vi "GUI Monitoring Graph Window.vi"(4 "Graph Unit":string, 6 "Window Title":string, 8 "BPM?":bool, 9 "Monitoring Queue Name":string, 10 "Selected Readings":u32[](array[numeric])=[0, 1, 2, 3, 4, 5, 6, 7, 8, 9, 10, 11, 12, 13, 14, 15, 16, 17, 18, 19, 20, 21, 22, 23, 24, 25, 26, 27, 28, 29, 30, 31, 32, 33, 34, 35], 11 "Variable Names":string[](array[string])=["ACH01B", "ACH02", "ACH03A", "ACH03B", "ACH04", "ACH05A", "ACH05B", "ACH06", "ACH07A", "ACH07B", "ACH08", "ACH09A", "ACH09B", "ACH10", "ACH11A", "ACH11B", "ACH12", "ACH01A"]) -> ()   [LabVIEW 2011, in "User Interface Window VIs.lvlib"]
uses:
  User Interface Window VIs.lvlib
  Types Definitions/Type Monitoring Sample.ctl
  <vilib>/Platform/TimedLoop/XDataNode/timing_clust.ctl
  <vilib>/Platform/TimedLoop/XDataNode/nitl_modes.ctl
  <vilib>/Platform/TimedLoop/XDataNode/wakeup.ctl
  <vilib>/express/express shared/transition.llb/Dynamic To Waveform Array.vi
  <vilib>/express/express signal manip/GetorSetDDTAttributes/Set DDT Attributes/SetT0.vi
  <vilib>/express/express shared/transition.llb/Waveform Array To Dynamic.vi
  <vilib>/Platform/TimedLoop/XDataNode/XDataNode.xnode
  <vilib>/express/express signal manip/GetorSetDDTAttributes/Set DDT Attributes/Set DDT Properties.xnode
  Common VIs.lvlib
  <vilib>/Platform/TimedLoop/XDataNode/XDNodeRunTimeDep.lvlib
  User Interface VIs.lvlib
  Type Definitions.lvlib
panel:
  out "Time Stamp on FOFB Controller":timestamp caption="Data/Hora Atual no\nControlador do FOFB"
  out "error out":errorcluster
  in  "All/None":bool=TRUE caption="Todos/Nenhum"
  out "Graph":dynamicdata(graph)=[{"t0"=timestamp(3440556827.6210413 s since 1904-01-01), "dt"=1.0, "Y"=[0.004733479817708333], "attributes"=variant("NI_ExpTimeStamp"=variant(timestamp timestamp(3440556827.6210413 s since 1904-01-01)))}, {"t0"=timestamp(3440556827.6210413 s since 1904-01-01), "dt"=1.0, "Y"=[0.004206909179687498], "attributes"=variant("NI_ExpTimeStamp"=variant(timestamp timestamp(3440556827.6210413 s since 1904-01-01)))}, {"t0"=timestamp(3440556827.6210413 s since 1904-01-01), "dt"=1.0, "Y"=[-10.43072509765625], "attributes"=variant("NI_ExpTimeStamp"=variant(timestamp timestamp(3440556827.6210413 s since 1904-01-01)))}, {"t0"=timestamp(3440556827.6210413 s since 1904-01-01), "dt"=1.0, "Y"=[-10.430725128173831], "attributes"=variant("NI_ExpTimeStamp"=variant(timestamp timestamp(3440556827.6210413 s since 1904-01-01)))}, {"t0"=timestamp(3440556827.6210413 s since 1904-01-01), "dt"=1.0, "Y"=[0.010971476236979166], "attributes"=variant("NI_ExpTimeStamp"=variant(timestamp timestamp(3440556827.6210413 s since 1904-01-01)))}, {"t0"=timestamp(3440556827.6210413 s since 1904-01-01), "dt"=1.0, "Y"=[0.01062655639648437], "attributes"=variant("NI_ExpTimeStamp"=variant(timestamp timestamp(3440556827.6210413 s since 1904-01-01)))}, {"t0"=timestamp(3440556827.6210413 s since 1904-01-01), "dt"=1.0, "Y"=[0.006206461588541667], "attributes"=variant("NI_ExpTimeStamp"=variant(timestamp timestamp(3440556827.6210413 s since 1904-01-01)))}, {"t0"=timestamp(3440556827.6210413 s since 1904-01-01), "dt"=1.0, "Y"=[0.0061141052246093735], "attributes"=variant("NI_ExpTimeStamp"=variant(timestamp timestamp(3440556827.6210413 s since 1904-01-01)))}, {"t0"=timestamp(3440556827.6210413 s since 1904-01-01), "dt"=1.0, "Y"=[-10.42022705078125], "attributes"=variant("NI_ExpTimeStamp"=variant(timestamp timestamp(3440556827.6210413 s since 1904-01-01)))}, {"t0"=timestamp(3440556827.6210413 s since 1904-01-01), "dt"=1.0, "Y"=[-10.42022705078125], "attributes"=variant("NI_ExpTimeStamp"=variant(timestamp timestamp(3440556827.6210413 s since 1904-01-01)))}, {"t0"=timestamp(3440556827.6210413 s since 1904-01-01), "dt"=1.0, "Y"=[-10.37188720703125], "attributes"=variant("NI_ExpTimeStamp"=variant(timestamp timestamp(3440556827.6210413 s since 1904-01-01)))}, {"t0"=timestamp(3440556827.6210413 s since 1904-01-01), "dt"=1.0, "Y"=[-10.37188720703125], "attributes"=variant("NI_ExpTimeStamp"=variant(timestamp timestamp(3440556827.6210413 s since 1904-01-01)))}, {"t0"=timestamp(3440556827.6210413 s since 1904-01-01), "dt"=1.0, "Y"=[0.0069844563802083336], "attributes"=variant("NI_ExpTimeStamp"=variant(timestamp timestamp(3440556827.6210413 s since 1904-01-01)))}, {"t0"=timestamp(3440556827.6210413 s since 1904-01-01), "dt"=1.0, "Y"=[0.007014038085937505], "attributes"=variant("NI_ExpTimeStamp"=variant(timestamp timestamp(3440556827.6210413 s since 1904-01-01)))}, {"t0"=timestamp(3440556827.6210413 s since 1904-01-01), "dt"=1.0, "Y"=[0.0], "attributes"=variant("NI_ExpTimeStamp"=variant(timestamp timestamp(3440556827.6210413 s since 1904-01-01)))}, {"t0"=timestamp(3440556827.6210413 s since 1904-01-01), "dt"=1.0, "Y"=[0.0], "attributes"=variant("NI_ExpTimeStamp"=variant(timestamp timestamp(3440556827.6210413 s since 1904-01-01)))}, {"t0"=timestamp(3440556827.6210413 s since 1904-01-01), "dt"=1.0, "Y"=[0.0], "attributes"=variant("NI_ExpTimeStamp"=variant(timestamp timestamp(3440556827.6210413 s since 1904-01-01)))}, {"t0"=timestamp(3440556827.6210413 s since 1904-01-01), "dt"=1.0, "Y"=[0.0], "attributes"=variant("NI_ExpTimeStamp"=variant(timestamp timestamp(3440556827.6210413 s since 1904-01-01)))}, {"t0"=timestamp(3440556827.6210413 s since 1904-01-01), "dt"=1.0, "Y"=[0.0], "attributes"=variant("NI_ExpTimeStamp"=variant(timestamp timestamp(3440556827.6210413 s since 1904-01-01)))}, {"t0"=timestamp(3440556827.6210413 s since 1904-01-01), "dt"=1.0, "Y"=[0.0], "attributes"=variant("NI_ExpTimeStamp"=variant(timestamp timestamp(3440556827.6210413 s since 1904-01-01)))}, {"t0"=timestamp(3440556827.6210413 s since 1904-01-01), "dt"=1.0, "Y"=[0.0], "attributes"=variant("NI_ExpTimeStamp"=variant(timestamp timestamp(3440556827.6210413 s since 1904-01-01)))}, {"t0"=timestamp(3440556827.6210413 s since 1904-01-01), "dt"=1.0, "Y"=[0.0], "attributes"=variant("NI_ExpTimeStamp"=variant(timestamp timestamp(3440556827.6210413 s since 1904-01-01)))}, {"t0"=timestamp(3440556827.6210413 s since 1904-01-01), "dt"=1.0, "Y"=[0.0], "attributes"=variant("NI_ExpTimeStamp"=variant(timestamp timestamp(3440556827.6210413 s since 1904-01-01)))}, {"t0"=timestamp(3440556827.6210413 s since 1904-01-01), "dt"=1.0, "Y"=[0.0], "attributes"=variant("NI_ExpTimeStamp"=variant(timestamp timestamp(3440556827.6210413 s since 1904-01-01)))}, {"t0"=timestamp(3440556827.6210413 s since 1904-01-01), "dt"=1.0, "Y"=[0.0], "attributes"=variant("NI_ExpTimeStamp"=variant(timestamp timestamp(3440556827.6210413 s since 1904-01-01)))}, {"t0"=timestamp(3440556827.6210413 s since 1904-01-01), "dt"=1.0, "Y"=[0.0], "attributes"=variant("NI_ExpTimeStamp"=variant(timestamp timestamp(3440556827.6210413 s since 1904-01-01)))}, {"t0"=timestamp(3440556827.6210413 s since 1904-01-01), "dt"=1.0, "Y"=[0.0], "attributes"=variant("NI_ExpTimeStamp"=variant(timestamp timestamp(3440556827.6210413 s since 1904-01-01)))}, {"t0"=timestamp(3440556827.6210413 s since 1904-01-01), "dt"=1.0, "Y"=[0.0], "attributes"=variant("NI_ExpTimeStamp"=variant(timestamp timestamp(3440556827.6210413 s since 1904-01-01)))}, {"t0"=timestamp(3440556827.6210413 s since 1904-01-01), "dt"=1.0, "Y"=[0.0], "attributes"=variant("NI_ExpTimeStamp"=variant(timestamp timestamp(3440556827.6210413 s since 1904-01-01)))}, {"t0"=timestamp(3440556827.6210413 s since 1904-01-01), "dt"=1.0, "Y"=[0.0], "attributes"=variant("NI_ExpTimeStamp"=variant(timestamp timestamp(3440556827.6210413 s since 1904-01-01)))}, {"t0"=timestamp(3440556827.6210413 s since 1904-01-01), "dt"=1.0, "Y"=[0.0], "attributes"=variant("NI_ExpTimeStamp"=variant(timestamp timestamp(3440556827.6210413 s since 1904-01-01)))}, {"t0"=timestamp(3440556827.6210413 s since 1904-01-01), "dt"=1.0, "Y"=[0.0], "attributes"=variant("NI_ExpTimeStamp"=variant(timestamp timestamp(3440556827.6210413 s since 1904-01-01)))}, {"t0"=timestamp(3440556827.6210413 s since 1904-01-01), "dt"=1.0, "Y"=[0.0], "attributes"=variant("NI_ExpTimeStamp"=variant(timestamp timestamp(3440556827.6210413 s since 1904-01-01)))}, {"t0"=timestamp(3440556827.6210413 s since 1904-01-01), "dt"=1.0, "Y"=[0.0], "attributes"=variant("NI_ExpTimeStamp"=variant(timestamp timestamp(3440556827.6210413 s since 1904-01-01)))}, {"t0"=timestamp(3440556827.6210413 s since 1904-01-01), "dt"=1.0, "Y"=[0.0], "attributes"=variant("NI_ExpTimeStamp"=variant(timestamp timestamp(3440556827.6210413 s since 1904-01-01)))}, {"t0"=timestamp(3440556827.6210413 s since 1904-01-01), "dt"=1.0, "Y"=[0.0], "attributes"=variant("NI_ExpTimeStamp"=variant(timestamp timestamp(3440556827.6210413 s since 1904-01-01)))}]
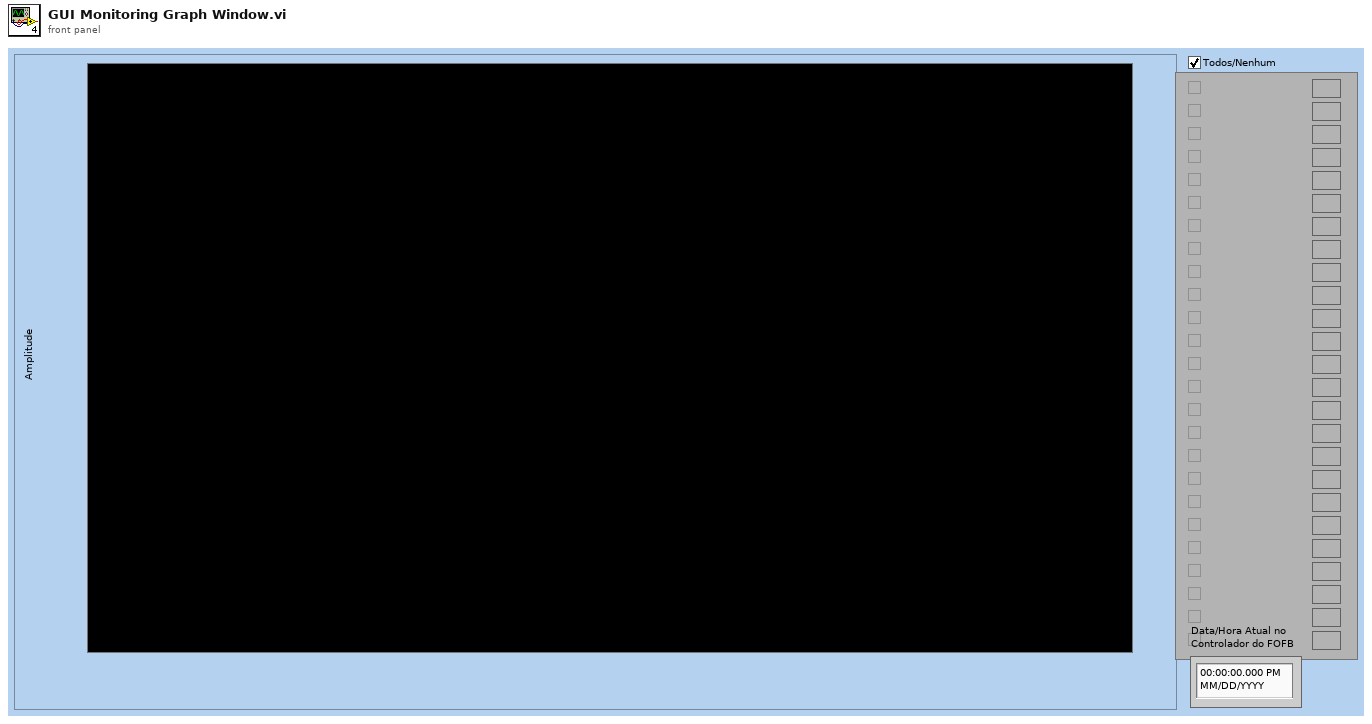
[diagram p1: front panel]
types:
  T1 = typedef "Semaphore RefNum" = refnum<k1>
  T2 = typedef "Type Definitions.lvlib/Type Monitoring Sample.ctl" = cluster{"Timestamp":timestamp, "Sample":dbl[]}
  T3 = enum32{"Invalid", "Standard", "Closed", "Hidden", "Minimized", "Maximized"}
  T4 = typedef "XDNodeRunTimeDep.lvlib/timing_clust.ctl" = cluster{"Expected End [f-1]":u64, "Actual End [f-1]":u64, "Finished Late? [f-1]":bool, "Expected End [i-1]":u64, "Actual End [i-1]":u64, "Finished Late? [i-1]":bool, "Expected Start [i]":u64, "Actual Start [i]":u64, "Expected Start [f]":u64, "Actual Start [f]":u64, "Source Name":string, "Structure Name":string, "Period":i64, "Deadline":i64, "Offset":i64, "Start":i64, "Priority":i32, "Timeout":i32, "Mode":T5, "Wakeup Reason":T6, "Error":errorcluster, "Source Type":string, "Secondary Source Type":string, "Global End Time":u64, "Global Start Time":u64, "Frame Duration":u64, "Iteration Duration":u64, "Assigned CPU":i32, "I/O Scan Engine Mode":u32}
  T5 = typedef "XDNodeRunTimeDep.lvlib/nitl_modes.ctl" = enum32{"No Change", "Process missed periods, maintain original phase", "Discard missed periods, maintain original phase", "Process missed periods, ignore original phase", "Discard missed periods, ignore original phase"}
  T6 = typedef "XDNodeRunTimeDep.lvlib/wakeup.ctl" = enum32{"Normal", "Aborted", "Asynchronous wakeup", "Timing source error", "Timed loop error", "Timeout"}
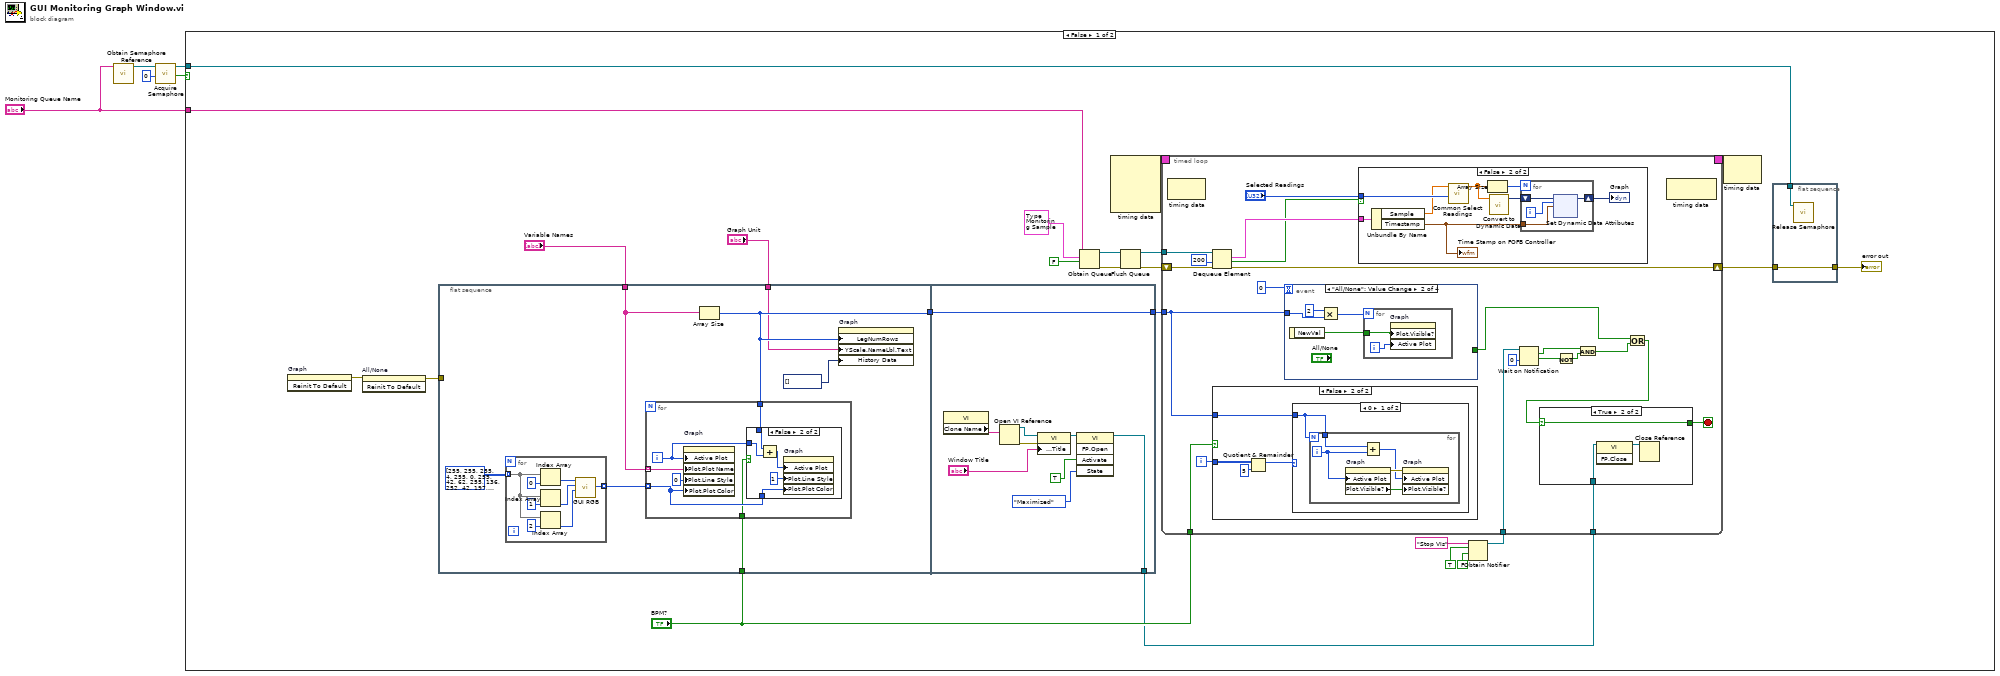
[diagram p0: block diagram]
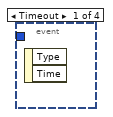
[diagram p7: hidden frame]
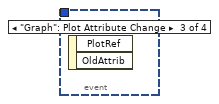
[diagram p8: hidden frame]
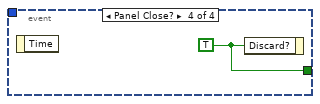
[diagram p9: hidden frame]
diagram:
  n1 = call <vilib>:"Obtain Semaphore Reference.vi"("name (unnamed)"="Monitoring Queue Name") -> ("semaphore"=w4:T1)  [unwired: 4 in, 2 out]
  n2 = call <vilib>:"Acquire Semaphore.vi"("ms timeout (-1)"=0, "semaphore"=w4) -> ("timed out"=w3:bool, "semaphore out"=w2:T1)  [unwired: 3 in, 1 out]
  n3 = case shown="False" w3 {
    tunnel: "Monitoring Queue Name" -> [w21 _]
    tunnel: w2 -> [w8 _]
    frame False {
      n4 = invoke on="Graph" class="WFChart (strict)" method="Reinit To Default"() -> (error out=w14:errorcluster)  [unwired: 3 in, 2 out]
      n5 = invoke on="All/None" class="Bool (strict)" method="Reinit To Default"(error in=w14) -> (error out=w13:errorcluster)  [unwired: 2 in, 2 out]
      n6 = flat-sequence {
        tunnel: w13 -> [_]
        tunnel: [w35] -> w27
        tunnel: "BPM?" -> [w34]
        tunnel: "Variable Names" -> [w33]
        tunnel: "Graph Unit" -> [w32]
        tunnel: [w66] -> w15
        tunnel: w27 -> [w66]
        tunnel: [w58] -> w9
        frame #0 {
          n7 = for {
            tunnel: [w46] -> w38 mode=indexing
            tunnel: u8[][] [[255, 255, 255], [4, 255, 0], [255, 42, 62], [255, 136, 252], [42, 197, 255], [187, 18, 255], [189, 227, 216], [255, 89, 137], [255, 0, 0], [210, 0, 220], [0, 120, 159], [89, 255, 167], [181, 219, 184], [220, 163, 0], [255, 127, 89], [110, 92, 130], [0, 11, 239], [255, 254, 0], [115, 25, 0], [210, 255, 113], [225, 100, 196], [225, 179, 18], [0, 115, 41], [115, 25, 0], [205, 89, 255]] -> [w45] mode=indexing
            n8 = Index Array(array=w45, index=0) -> (element=w44:u8)
            n9 = Index Array(array=w45, index=1) -> (element=w43:u8)
            n10 = Index Array(array=w45, index=2) -> (element=w42:u8)
            n11 = call "GUI RGB.vi"("Blue"=w42, "Green"=w43, "Red"=w44) -> ("result"=w46:u32)  [unwired: 8 in]
          }
          n12 = Array Size(array=w33) -> (size(s)=w35:i32)
          n13 = for {
            tunnel: w33 -> [w52] mode=indexing
            tunnel: w35 -> [w49]
            tunnel: w38 -> [w48] mode=indexing
            tunnel: w34 -> [w47]
            i -> [w50]
            n14 = property on="Graph" class="WFChart (strict)"("Active Plot"=w50, "Plot.Plot Name"=w52, "Plot.Line Style"=u8 0, "Plot.Plot Color"=w48) -> ()  [unwired: 2 in, 2 out]
            n15 = case shown="False" w47 {
              tunnel: w50 -> [_ w57]
              tunnel: w49 -> [_ w55]
              tunnel: w48 -> [_ w53]
              frame True {
              }
              frame False {
                n16 = Add(x=w55, y=w57) -> (x+y=w56:i32)
                n17 = property on="Graph" class="WFChart (strict)"("Active Plot"=w56, "Plot.Line Style"=u8 1, "Plot.Plot Color"=w53) -> ()  [unwired: 2 in, 2 out]
              }
            }
          }
          n18 = property on="Graph" class="WFChart (strict)"("LegNumRows"=w35, "YScale.NameLbl.Text"=w32, "History Data"=dynamicdata[] []) -> ()  [unwired: 2 in, 2 out]
        }
        frame #1 {
          n19 = property class="VI"() -> ("Clone Name"=w62:string)  [unwired: 2 in, 2 out]
          n20 = Open VI Reference(vi path=w62) -> (vi reference=w65:refnum<vi>, error out=w63:errorcluster)  [unwired: 5 in]
          n21 = property class="VI"(reference=w65, error in=w63, "Front Panel.Title"="Window Title") -> (reference out=w61:refnum<vi>)  [unwired: 1 out]
          n22 = invoke class="VI" method="FP.Open"(reference=w61, "Activate"=TRUE ("Activate?"), "State"=T3."Maximized") -> (reference out=w58:refnum<vi>)  [unwired: 2 in, 4 out]
        }
      }
      n23 = Obtain Queue(name (unnamed)=w21, element data type=T2 {"Timestamp"=timestamp(0 s since 1904-01-01), "Sample"=[]} ("Monitoring Sample"), create if not found? (T)=FALSE) -> (queue out=w22:refnum<queue>, error out=w20:errorcluster)  [unwired: 2 in, 1 out]
      n24 = node-c288() -> (w29:T4)  [unwired: 4 in]
      n25 = Flush Queue(queue=w22, error in (no error)=w20) -> (queue out=w25:refnum<queue>, error out=w26:errorcluster)  [unwired: 1 out]
      n26 = Obtain Notifier(name (unnamed)="Stop VIs", notification data type=TRUE, create if not found? (T)=FALSE) -> (notifier out=w16:refnum<notifier>)  [unwired: 1 in, 2 out]
      n27 = timed-loop {
        timing: w29 -> [_]
        timing-out: [_] -> w28
        tunnel: w25 -> [w79]
        tunnel: w15 -> [w80]
        shift-right: [w84] -> w7
        shift-left: w26 -> [w87]
        tunnel: w16 -> [w73]
        tunnel: "BPM?" -> [w69]
        tunnel: w9 -> [w67]
        i -> [w86]
        stop <- w74 stop-if-true
        n28 = node-c288() -> ()  [unwired: 1 in, 1 out]
        n29 = Dequeue Element(queue=w79, timeout in ms (-1)=200, error in (no error)=w87) -> (element=w81:T2, timed out?=w68:bool, error out=w84:errorcluster)  [unwired: 1 out]
        n30 = case shown="False" w69 {
          tunnel: w86 -> [_ w116]
          tunnel: w80 -> [_ w113]
          frame True {
          }
          frame False {
            n31 = Quotient & Remainder(x=w116, y=5) -> (x-y*floor(x/y)=w114:i32)  [unwired: 1 out]
            n32 = case shown="0" w114 {
              tunnel: w113 -> [w117 _]
              frame 0 {
                n33 = for {
                  N: w117 -> [_]
                  tunnel: w117 -> [w118]
                  i -> [w119]
                  n34 = property on="Graph" class="WFChart (strict)"("Active Plot"=w119) -> (error out=w122:errorcluster, "Plot.Visible?"=w120:bool)  [unwired: 2 in, 1 out]
                  n35 = Add(x=w118, y=w119) -> (x+y=w121:i32)
                  n36 = property on="Graph" class="WFChart (strict)"(error in=w122, "Active Plot"=w121, "Plot.Visible?"=w120) -> ()  [unwired: 1 in, 2 out]
                }
              }
              frame 1, Default {
              }
            }
          }
        }
        n37 = event shown="[1] \"All/None\": Value Change" {
          selector: _ -> [_ _ _ _]
          dyn-events: _ -> [_ _ _ _]
          timeout: 0 -> [_ _ _ _]
          tunnel: [_ _ _ w133] -> w70
          tunnel: w80 -> [_ w127 _ _]
          event Timeout {
            n38 = event-data() -> ()  [unwired: 1 in, 2 out]
          }
          event "All/None": Value Change {
            n39 = event-data() -> ("NewVal"=w130:bool)  [unwired: 1 in]
            n40 = Multiply(x=2, y=w127) -> (x*y=w128:i32)
            n41 = for {
              N: w128 -> [_]
              tunnel: w130 -> [w131]
              i -> [w132]
              n42 = property on="Graph" class="WFChart (strict)"("Plot.Visible?"=w131, "Active Plot"=w132) -> ()  [unwired: 2 in, 2 out]
            }
          }
          event "Graph": Plot Attribute Change {
            n43 = event-data() -> ()  [unwired: 1 in, 2 out]
          }
          event Panel Close? {
            w133 = TRUE
            n44 = event-data() -> ()  [unwired: 1 in, 1 out]
            n45 = event-data("Discard?"=w133) -> ()  [unwired: 1 in, 1 out]
          }
        }
        n46 = case shown="False" w68 {
          tunnel: "Selected Readings" -> [_ w92]
          tunnel: w81 -> [_ w91]
          frame True {
          }
          frame False {
            n47 = Unbundle By Name(w91) -> ("Sample"=w90:dbl[], "Timestamp"=w89:timestamp)
            "Time Stamp on FOFB Controller" <- w89
            n48 = call "Common Select Readings.vi"("Selected Readings"=w92, "Readings"=w90) -> ("Readings Subset"=w93:dbl[])  [unwired: 9 in]
            n49 = Array Size(array=w93) -> (size(s)=w95:i32)
            n50 = call "Convert to Dynamic Data"("Array"=w93) -> ("Dynamic Data Type"=w94:dynamicdata)  [unwired: 3 in]
            n51 = for {
              N: w95 -> [_]
              shift-right: [w99] -> w88
              shift-left: w94 -> [w97]
              tunnel: w89 -> [w96]
              i -> [w98]
              n52 = xnode ("Set Dynamic Data Attributes")("Signals In"=w97, "Signal Index"=w98, "Timestamp"=w96) -> ("Signals Out"=w99:dynamicdata)  [unwired: 1 in, 1 out]
            }
            "Graph" <- w88
          }
        }
        n53 = Wait on Notification(notifier=w73, timeout in ms (-1)=0) -> (notification=w75:bool, timed out?=w77:bool)  [unwired: 2 in, 2 out]
        n54 = Not(x=w77) -> (.not. x?=w76:bool)
        n55 = And(x=w75, y=w76) -> (x .and. y?=w71:bool)
        n56 = Or(x=w70, y=w71) -> (x .or. y?=w72:bool)
        n57 = case shown="True" w72 {
          selector: w72 -> [w123 w126]
          tunnel: [w123 w126] -> w74
          tunnel: w67 -> [_ w124]
          frame False {
          }
          frame True {
            n58 = invoke class="VI" method="FP.Close"(reference=w124) -> (reference out=w125:refnum<vi>)  [unwired: 2 in, 2 out]
            n59 = Close Reference(reference=w125) -> ()  [unwired: 1 in, 1 out]
          }
        }
        n60 = node-c288() -> ()  [unwired: 1 in, 1 out]
      }
      n61 = node-c288(w28) -> ()  [unwired: 1 out]
      n62 = flat-sequence {
        tunnel: w8 -> [w31]
        tunnel: w7 -> [w30]
        tunnel: [w30] -> w6
        frame #0 {
          n63 = call <vilib>:"Release Semaphore.vi"("semaphore"=w31) -> ()  [unwired: 5 in, 2 out]
        }
      }
      "error out" <- w6
    }
    frame True {
    }
  }
